vi "Agilent VNA Fetch Data.vi"(4 "Trace":i8=1 min=1 max=99 step=1, 6 "Channel":i8=1 min=1 max=99 step=1, 7 "Agilent VNA":T2, 8 "error in (no error)":errorcluster, 9 "Formatted Data?":bool, 10 "Data to Read (Data)":enum16{"Data", "Memory"}(ring), 11 "VISA Resource Name":refnum<visa-resource-name>) -> (0 "error out":errorcluster, 1 "Display Format":T1, 2 "Data (real+imag)":cdb[](array[numeric]), 3 "dup VISA Resource Name":refnum<visa-resource-name>)   [LabVIEW 2011]
doc: "It is recommended that you hold off triggers before running this VI as the HP8753 tends to \"hang\" if data is read while measurements are being taken.\n\n This VI is used to collect and display data generated by the HP8753 Network Analyzer. The VI can display error-corrected data, error-corrected trace memory, fully formatted data and memory traces. For further information on these types of data see Processsing Chain figure in the HPIB programming note. When the data type is a formatted data, the instruments screen will change to reflect what is being displayed, eg. selecting \"formatted memory\" changes the display to \"MEMORY\".\n\n The data values shown depend upon the data type and the measurement format. If the data type is \"error-corrected data\" or \"error-corrected trace memory\" and/or the measurement format is \"Smith chart\" or \"polar\", the data values are real,imaginary pairs. Otherwise the data values are stimulus,response pairs. These pairs correspond to what is shown in the graphical display.\n\n Data can also be saved to a file with this VI. When saving a file, the stimulus is always shown. The real,imaginary components or the response value are also shown depending upon the data type and the measurement format. \n\n No units are shown on the VI front panel or in the data file. All units are basic units of Hz, dB, seconds, ohms, etc. The \"saved data comments\" control should be used for any special information such as the measurement format, averaging and smoothing information, etc.\n\n Whether or not data is saved and whether the output is in real,imaginary pairs or stimulus,response parirs affects the speed of this VI. When data is saved to a file and/or when data is in stimulus,response pairs, requires the reading of the stimulus values which slows the VI down. The fastest reads are done when the data type is \"error-corrected data\" or \"error-corrected trace memory\" and/or the measurement format is \"Smith chart\" or \"polar\" and data is not being saved to a file.\n\n This VI sets the format, ie. linear or logarithmic, depending upon the sweep type. \n\nFYI - Originally this VI was written without considering the stimulus values. In most case this would be fine for display purposes as the point number could be used for the X value as most sweeps are evenly spaced. This is not the case with frequency list sweeps which can have big gaps in the sweep. For this reason the stimulus value is read (at least in the cases explained above) to make the LabVIEW display match what is display on the instrument's display."
uses:
  TypeDefs/Agilent VNA Instrument Info.ctl
  tests/S Parameter/TypeDefs/SP Measurement Format.ctl
panel:
  out "#data points":i16
  out "bytes to read\n(divide this number\nby 6 bytes per point\nto get # points for\na sanity check)":i16
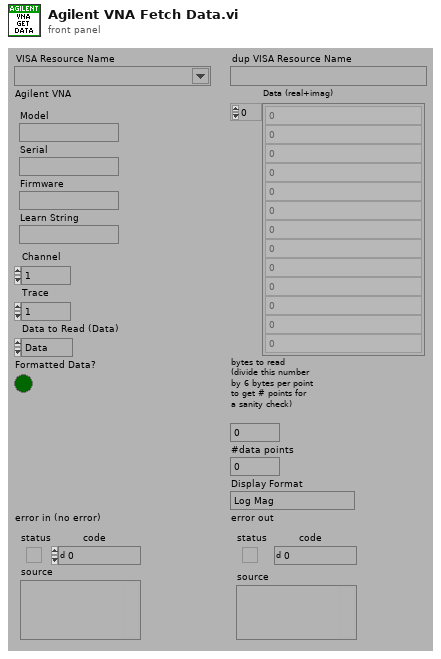
[diagram p1: front panel]
types:
  T1 = typedef "SP Measurement Format.ctl" = enum32{"Log Mag", "Phase", "Delay", "Smith (R+jX)", "Polar (Re/Im)", "Linear Mag", "SWR", "Real", "Imaginary", "Smith (Lin/Phase)", "Smith (Log/Phase)", "Smith (Real/Imag)", "Smith (G+jB)", "Polar (Lin/Phase)", "Polar (Log/Phase)", "Expanded Phase", "Positive Phase", "Inverted Smith", "Unwrapped Phase", "Power Out", "Power In", "Linear Mag/Phase", "Log Mag/Phase", "Real/Imaginary"}
  T2 = typedef "Agilent VNA Instrument Info.ctl" = cluster{"Model":string, "Serial":string, "Firmware":string, "Learn String":string}
  T3 = typedef "Agilent VNA Model.ctl" = enum16{"Not Supported", "8510X", "8719X", "8720X", "8722X", "8753X", "ENA", "PNA", "Field Fox"}
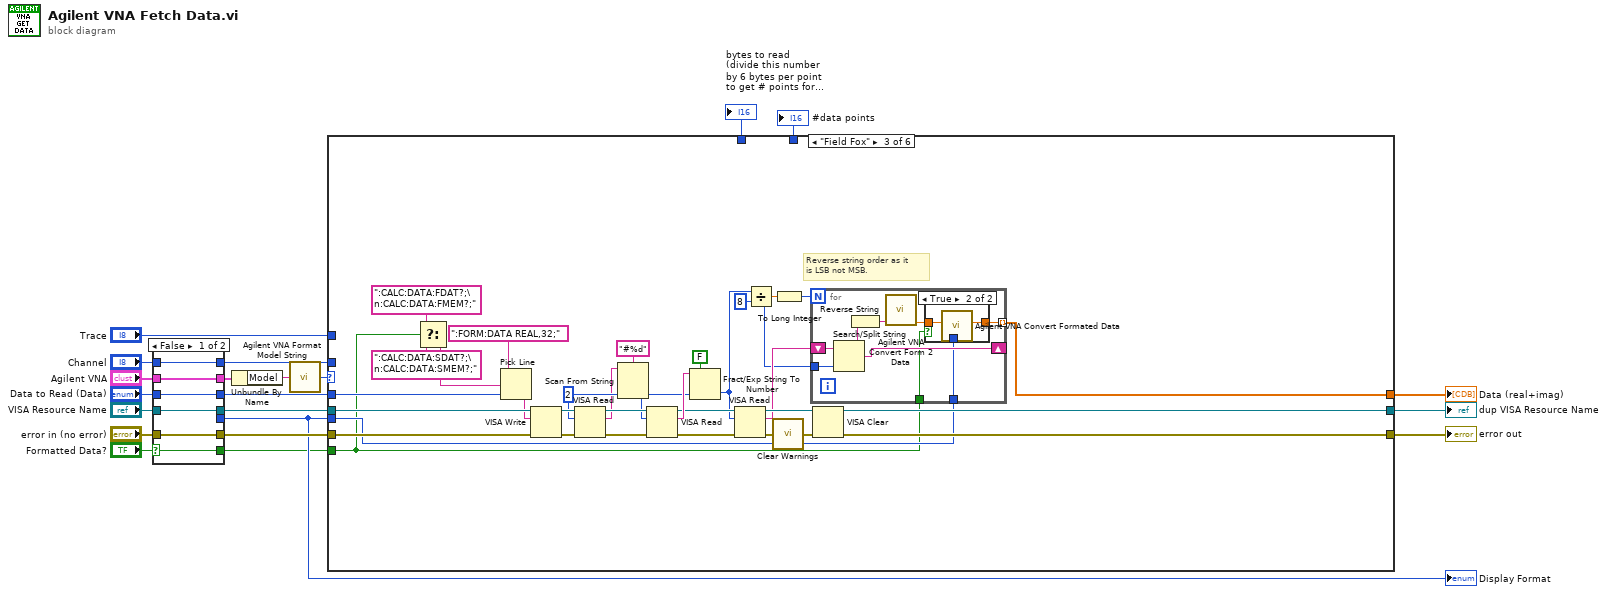
[diagram p0: block diagram]
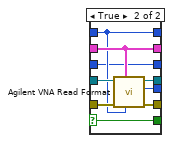
[diagram p2: hidden frame]
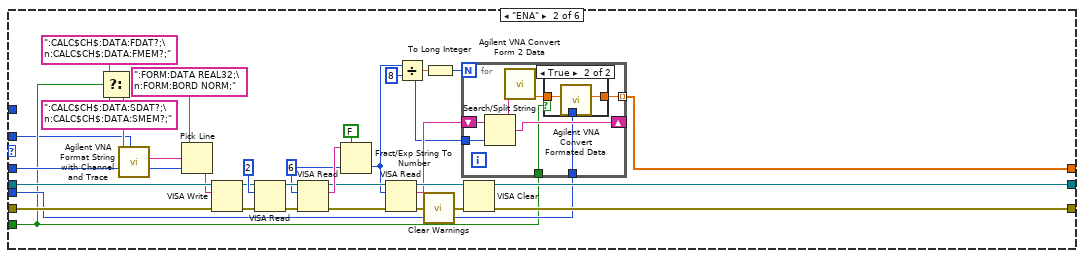
[diagram p4: hidden frame]
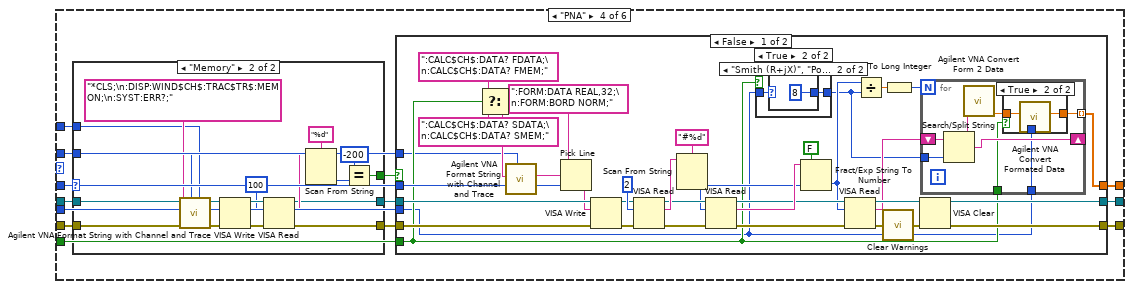
[diagram p7: hidden frame]
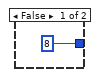
[diagram p9: hidden frame]
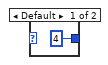
[diagram p10: hidden frame]
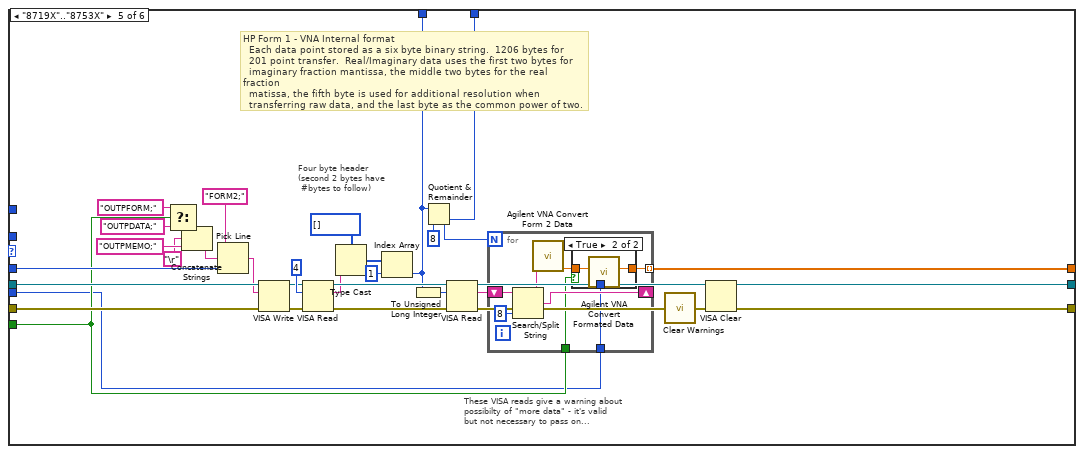
[diagram p13: hidden frame]
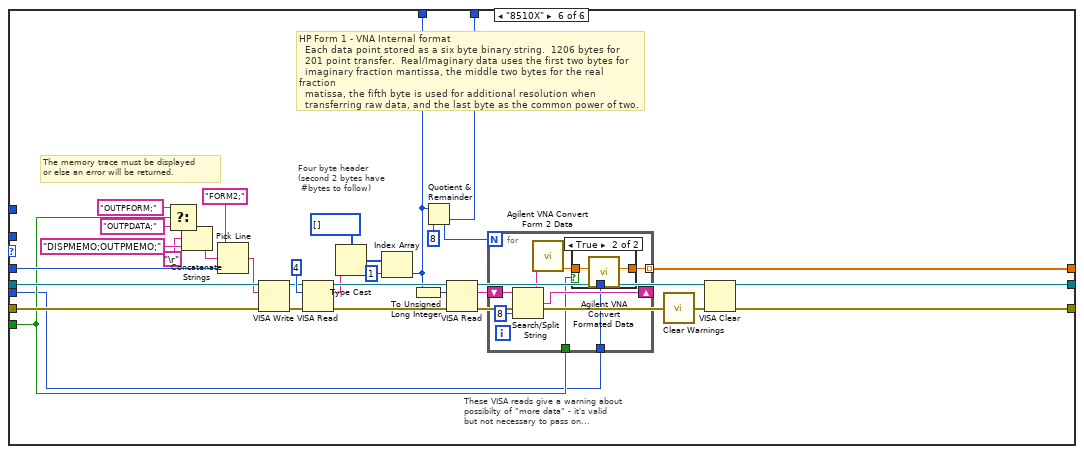
[diagram p15: hidden frame]
diagram:
  n1 = case shown="False" "Formatted Data?" {
    selector: "Formatted Data?" -> [w22 w28]
    tunnel: "error in (no error)" -> [w27 w36]
    tunnel: "VISA Resource Name" -> [w26 w35]
    tunnel: [w26 w34] -> w16
    tunnel: [w27 w33] -> w15
    tunnel: "Agilent VNA" -> [w25 w32]
    tunnel: "Channel" -> [w24 w31]
    tunnel: [w25 w32] -> w2
    tunnel: [w24 w31] -> w12
    tunnel: "Data to Read (Data)" -> [w23 w30]
    tunnel: [w23 w30] -> w10
    tunnel: [_ w29] -> w9
    tunnel: [w22 w28] -> w7
    frame False {
    }
    frame True {
      n2 = call "Agilent VNA Read Format.vi"("Channel"=w31, "Agilent VNA"=w32, "error in (no error)"=w36, "VISA Resource Name"=w35) -> ("error out"=w33:errorcluster, "Display Format"=w29:T1, "dup VISA Resource Name"=w34:refnum<visa-resource-name>)  [unwired: 5 out]
    }
  }
  "Display Format" <- w9
  n3 = Unbundle By Name(w2) -> ("Model"=w1:string)
  n4 = call "Agilent VNA Format Model String.vi"("Model"=w1) -> ("Model"=w19:T3)
  n5 = case shown="\"Field Fox\"" w19 {
    tunnel: w16 -> [w38 w70 w116 w137 w244 w289]
    tunnel: w15 -> [w37 w68 w114 w136 w240 w285]
    tunnel: [w37 w54 w108 w141 w216 w262] -> w3
    tunnel: [_ w48 w107 w140 w224 w269] -> w21
    tunnel: [w38 w55 w109 w142 w217 w261] -> w20
    tunnel: w10 -> [_ w58 w110 w133 w235 w280]
    tunnel: w12 -> [_ w41 _ w132 _ _]
    tunnel: w9 -> [_ w44 w104 w138 w222 w267]
    tunnel: w7 -> [_ w43 w103 w139 w223 w268]
    tunnel: [_ _ _ _ w220 w266] -> w6
    tunnel: [_ _ _ _ w221 w265] -> w5
    tunnel: "Trace" -> [_ _ _ w130 _ _]
    frame "Not Supported" {
    }
    frame "ENA" {
      w42 = 8
      w59 = u32 6
      n6 = Select(t=":CALC$CH$:DATA:FDAT?;\n:CALC$CH$:DATA:FMEM?;" ("String"), s=w43, f=":CALC$CH$:DATA:SDAT?;\n:CALC$CH$:DATA:SMEM?;" ("String")) -> (s? t:f=w45:string)
      n7 = call "Agilent VNA Format String with Channel and Trace.vi"("Channel"=w41, "String"=w45) -> ("String Out"=w66:string)  [unwired: 1 in, 6 out]
      n8 = Pick Line(string ("")=":FORM:DATA REAL32;\n:FORM:BORD NORM;" ("String"), multi-line string=w66, line index=w58) -> (output string=w64:string)
      n9 = VISA Write(VISA resource name=w70, write buffer=w64, error in (no error)=w68) -> (VISA resource name out=w69:refnum<visa-resource-name>, error out=w67:errorcluster)  [unwired: 1 out]
      n10 = VISA Read(VISA resource name=w69, byte count=u32 2, error in (no error)=w67) -> (VISA resource name out=w63:refnum<visa-resource-name>, error out=w62:errorcluster)  [unwired: 2 out]
      n11 = VISA Read(VISA resource name=w63, byte count=w59, error in (no error)=w62) -> (VISA resource name out=w53:refnum<visa-resource-name>, read buffer=w60:string, error out=w52:errorcluster)  [unwired: 1 out]
      n12 = Fract/Exp String To Number(use system decimal point (T)=FALSE, string=w60, default (0 dbl)=w59) -> (number=w51:u32)  [unwired: 2 out]
      n13 = VISA Read(VISA resource name=w53, byte count=w51, error in (no error)=w52) -> (VISA resource name out=w50:refnum<visa-resource-name>, read buffer=w49:string, error out=w40:errorcluster)  [unwired: 1 out]
      n14 = Divide(x=w51, y=w42) -> (x/y=w57:dbl)
      n15 = call "Clear Warnings.vi"("error in (no error)"=w40) -> ("error out"=w39:errorcluster)
      n16 = To Long Integer(number=w57) -> (32bit integer=w56:i32)
      n17 = for {
        N: w56 -> [_]
        shift-right: [w77] -> _
        shift-left: w49 -> [w78]
        tunnel: [w75] -> w48 mode=indexing
        tunnel: w44 -> [w74]
        tunnel: w43 -> [w73]
        tunnel: w42 -> [w72]
        n18 = Search/Split String(string=w78, offset (0)=w72) -> (substring before match=w76:string, match + rest of string=w77:string)  [unwired: 2 out]
        n19 = call "Agilent VNA Convert Form 2 Data.vi"("Raw Data Point"=w76) -> ("Number"=w79:cdb)  [unwired: 10 out]
        n20 = case shown="True" w73 {
          tunnel: w79 -> [w80 w82]
          tunnel: [w80 w81] -> w75
          tunnel: w74 -> [_ w83]
          frame False {
          }
          frame True {
            n21 = call "Agilent VNA Convert Formated Data.vi"("Display Format"=w83, "Number"=w82) -> ("Number"=w81:cdb)  [unwired: 9 out]
          }
        }
      }
      n22 = VISA Clear(VISA resource name=w50, error in (no error)=w39) -> (VISA resource name out=w55:refnum<visa-resource-name>, error out=w54:errorcluster)
    }
    frame "Field Fox" {
      w91 = 8
      w86 = u32 2
      # "Reverse string order as it\nis LSB not MSB."
      n23 = Select(t=":CALC:DATA:FDAT?;\n:CALC:DATA:FMEM?;" ("String"), s=w103, f=":CALC:DATA:SDAT?;\n:CALC:DATA:SMEM?;" ("String")) -> (s? t:f=w102:string)
      n24 = Pick Line(string ("")=":FORM:DATA REAL,32;" ("String"), multi-line string=w102, line index=w110) -> (output string=w111:string)
      n25 = VISA Write(VISA resource name=w116, write buffer=w111, error in (no error)=w114) -> (VISA resource name out=w115:refnum<visa-resource-name>, error out=w113:errorcluster)  [unwired: 1 out]
      n26 = VISA Read(VISA resource name=w115, byte count=w86, error in (no error)=w113) -> (VISA resource name out=w101:refnum<visa-resource-name>, read buffer=w84:string, error out=w100:errorcluster)  [unwired: 1 out]
      n27 = Scan From String(format string="#%d", input string=w84, default 1=w86) -> (output 1=w85:u32)  [unwired: 2 in, 3 out]
      n28 = VISA Read(VISA resource name=w101, byte count=w85, error in (no error)=w100) -> (VISA resource name out=w96:refnum<visa-resource-name>, read buffer=w99:string, error out=w95:errorcluster)  [unwired: 1 out]
      n29 = Fract/Exp String To Number(use system decimal point (T)=FALSE, string=w99, default (0 dbl)=w85) -> (number=w94:u32)  [unwired: 2 out]
      n30 = VISA Read(VISA resource name=w96, byte count=w94, error in (no error)=w95) -> (VISA resource name out=w93:refnum<visa-resource-name>, read buffer=w92:string, error out=w90:errorcluster)  [unwired: 1 out]
      n31 = Divide(x=w94, y=w91) -> (x/y=w98:dbl)
      n32 = call "Clear Warnings.vi"("error in (no error)"=w90) -> ("error out"=w89:errorcluster)
      n33 = To Long Integer(number=w98) -> (32bit integer=w97:i32)
      n34 = for {
        N: w97 -> [_]
        shift-right: [w123] -> _
        shift-left: w92 -> [w124]
        tunnel: [w122] -> w107 mode=indexing
        tunnel: w104 -> [w121]
        tunnel: w103 -> [w120]
        tunnel: w91 -> [w119]
        n35 = Search/Split String(string=w124, offset (0)=w119) -> (substring before match=w118:string, match + rest of string=w123:string)  [unwired: 2 out]
        n36 = Reverse String(1:w118) -> (0:w117:string)
        n37 = call "Agilent VNA Convert Form 2 Data.vi"("Raw Data Point"=w117) -> ("Number"=w125:cdb)  [unwired: 10 out]
        n38 = case shown="True" w120 {
          tunnel: w125 -> [w126 w128]
          tunnel: [w126 w127] -> w122
          tunnel: w121 -> [_ w129]
          frame False {
          }
          frame True {
            n39 = call "Agilent VNA Convert Formated Data.vi"("Display Format"=w129, "Number"=w128) -> ("Number"=w127:cdb)  [unwired: 9 out]
          }
        }
      }
      n40 = VISA Clear(VISA resource name=w93, error in (no error)=w89) -> (VISA resource name out=w109:refnum<visa-resource-name>, error out=w108:errorcluster)
    }
    frame "PNA" {
      n41 = case shown="\"Memory\"" w133 {
        tunnel: w137 -> [w144 w160]
        tunnel: w136 -> [w143 w159]
        tunnel: [w144 w151] -> w135
        tunnel: [w143 w150] -> w134
        tunnel: w132 -> [_ w146]
        tunnel: [_ w147] -> w131
        tunnel: w130 -> [_ w145]
        frame "Data", Default {
        }
        frame "Memory" {
          n42 = call "Agilent VNA Format String with Channel and Trace.vi"("Trace"=w145, "Channel"=w146, "String"="*CLS;\n:DISP:WIND$CH$:TRAC$TR$:MEM ON;\n:SYST:ERR?;") -> ("String Out"=w157:string)  [unwired: 6 out]
          n43 = VISA Write(VISA resource name=w160, write buffer=w157, error in (no error)=w159) -> (VISA resource name out=w156:refnum<visa-resource-name>, error out=w155:errorcluster)  [unwired: 1 out]
          n44 = VISA Read(VISA resource name=w156, byte count=u32 100, error in (no error)=w155) -> (VISA resource name out=w151:refnum<visa-resource-name>, read buffer=w153:string, error out=w150:errorcluster)  [unwired: 1 out]
          n45 = Scan From String(format string="%d", input string=w153) -> (output 1=w149:i32)  [unwired: 2 in, 4 out]
          n46 = Equal?(x=-200, y=w149) -> (x = y?=w147:bool)
        }
      }
      n47 = case shown="False" w131 {
        tunnel: w135 -> [w194 w213]
        tunnel: w134 -> [w192 w214]
        tunnel: w133 -> [w185 _]
        tunnel: [w182 w213] -> w142
        tunnel: [w181 w214] -> w141
        tunnel: w132 -> [w163 _]
        tunnel: [w175 _] -> w140
        tunnel: w139 -> [w166 _]
        tunnel: w138 -> [w165 _]
        frame False {
          n48 = Select(t=":CALC$CH$:DATA? FDATA;\n:CALC$CH$:DATA? FMEM;" ("String"), s=w166, f=":CALC$CH$:DATA? SDATA;\n:CALC$CH$:DATA? SMEM;" ("String")) -> (s? t:f=w172:string)
          n49 = call "Agilent VNA Format String with Channel and Trace.vi"("Channel"=w163, "String"=w172) -> ("String Out"=w190:string)  [unwired: 1 in, 6 out]
          n50 = Pick Line(string ("")=":FORM:DATA REAL,32;\n:FORM:BORD NORM;" ("String"), multi-line string=w190, line index=w185) -> (output string=w188:string)
          n51 = VISA Write(VISA resource name=w194, write buffer=w188, error in (no error)=w192) -> (VISA resource name out=w193:refnum<visa-resource-name>, error out=w191:errorcluster)  [unwired: 1 out]
          n52 = VISA Read(VISA resource name=w193, byte count=u32 2, error in (no error)=w191) -> (VISA resource name out=w168:refnum<visa-resource-name>, read buffer=w171:string, error out=w169:errorcluster)  [unwired: 1 out]
          n53 = Scan From String(format string="#%d", input string=w171) -> (output 1=w167:i32)  [unwired: 2 in, 4 out]
          n54 = VISA Read(VISA resource name=w168, byte count=w167, error in (no error)=w169) -> (VISA resource name out=w180:refnum<visa-resource-name>, read buffer=w186:string, error out=w179:errorcluster)  [unwired: 1 out]
          n55 = case shown="True" w166 {
            tunnel: w165 -> [_ w198]
            tunnel: [8 w197] -> w164
            frame False {
            }
            frame True {
              n56 = case shown="\"Smith (R+jX)\", \"Polar (Re/Im)\", \"Smith (Lin/Phase)\"..\"Polar (Log/Phase)\", \"Inverted Smith\"" w198 {
                tunnel: [4 8] -> w197
                frame Default {
                }
                frame "Smith (R+jX)", "Polar (Re/Im)", "Smith (Lin/Phase)".."Polar (Log/Phase)", "Inverted Smith" {
                }
              }
            }
          }
          n57 = Fract/Exp String To Number(use system decimal point (T)=FALSE, string=w186, default (0 dbl)=w167) -> (number=w178:i32)  [unwired: 2 out]
          n58 = VISA Read(VISA resource name=w180, byte count=w178, error in (no error)=w179) -> (VISA resource name out=w177:refnum<visa-resource-name>, read buffer=w176:string, error out=w162:errorcluster)  [unwired: 1 out]
          n59 = Divide(x=w178, y=w164) -> (x/y=w184:dbl)
          n60 = call "Clear Warnings.vi"("error in (no error)"=w162) -> ("error out"=w161:errorcluster)
          n61 = To Long Integer(number=w184) -> (32bit integer=w183:i32)
          n62 = VISA Clear(VISA resource name=w177, error in (no error)=w161) -> (VISA resource name out=w182:refnum<visa-resource-name>, error out=w181:errorcluster)
          n63 = for {
            N: w183 -> [_]
            shift-right: [w206] -> _
            shift-left: w176 -> [w207]
            tunnel: [w204] -> w175 mode=indexing
            tunnel: w165 -> [w203]
            tunnel: w166 -> [w202]
            tunnel: w164 -> [w201]
            n64 = Search/Split String(string=w207, offset (0)=w201) -> (substring before match=w205:string, match + rest of string=w206:string)  [unwired: 2 out]
            n65 = call "Agilent VNA Convert Form 2 Data.vi"("Raw Data Point"=w205) -> ("Number"=w208:cdb)  [unwired: 10 out]
            n66 = case shown="True" w202 {
              tunnel: w208 -> [w209 w211]
              tunnel: [w209 w210] -> w204
              tunnel: w203 -> [_ w212]
              frame False {
              }
              frame True {
                n67 = call "Agilent VNA Convert Formated Data.vi"("Display Format"=w212, "Number"=w211) -> ("Number"=w210:cdb)  [unwired: 9 out]
              }
            }
          }
        }
        frame True {
        }
      }
    }
    frame "8719X".."8753X" {
      # "These VISA reads give a warning about\npossibilty of \"more data\" - it's valid\nbut not necessary to pass on..."
      # "Four byte header\n(second 2 bytes have\n #bytes to follow)"
      # "HP Form 1 - VNA Internal format\n  Each data point stored as a six byte binary string.  1206 bytes for\n  201 point transfer.  Real/Imaginary data uses the first two bytes for\n  imaginary fraction mantissa, the middle two bytes for the real fraction\n  matissa, the fifth byte is used for additional resolution when\n  transferring raw data, and the last byte as the common power of two."
      n68 = Select(t="OUTPFORM;", s=w223, f="OUTPDATA;") -> (s? t:f=w226:string)
      n69 = Concatenate Strings(w226, "\r", "OUTPMEMO;") -> (w230:string)
      n70 = Pick Line(string ("")="FORM2;", multi-line string=w230, line index=w235) -> (output string=w234:string)
      n71 = VISA Write(VISA resource name=w244, write buffer=w234, error in (no error)=w240) -> (VISA resource name out=w233:refnum<visa-resource-name>, error out=w232:errorcluster)  [unwired: 1 out]
      n72 = VISA Read(VISA resource name=w233, byte count=u32 4, error in (no error)=w232) -> (VISA resource name out=w246:refnum<visa-resource-name>, read buffer=w238:string, error out=w245:errorcluster)  [unwired: 1 out]
      n73 = Type Cast(type=i16[] [], x=w238) -> (*(type *) &x=w237:i16[])
      n74 = Index Array(array=w237, index=1) -> (element=w221:i16)
      n75 = To Unsigned Long Integer(number=w221) -> (unsigned 32bit integer=w242:u32)
      n76 = Quotient & Remainder(x=w221, y=i16 8) -> (floor(x/y)=w220:i16)  [unwired: 1 out]
      n77 = VISA Read(VISA resource name=w246, byte count=w242, error in (no error)=w245) -> (VISA resource name out=w219:refnum<visa-resource-name>, read buffer=w239:string, error out=w215:errorcluster)  [unwired: 1 out]
      n78 = for {
        N: w220 -> [_]
        shift-right: [w254] -> _
        shift-left: w239 -> [w255]
        tunnel: [w250] -> w224 mode=indexing
        tunnel: w223 -> [w249]
        tunnel: w222 -> [w248]
        n79 = Search/Split String(string=w255, offset (0)=8) -> (substring before match=w252:string, match + rest of string=w254:string)  [unwired: 2 out]
        n80 = call "Agilent VNA Convert Form 2 Data.vi"("Raw Data Point"=w252) -> ("Number"=w251:cdb)  [unwired: 10 out]
        n81 = case shown="True" w249 {
          tunnel: w251 -> [w256 w258]
          tunnel: [w256 w257] -> w250
          tunnel: w248 -> [_ w259]
          frame False {
          }
          frame True {
            n82 = call "Agilent VNA Convert Formated Data.vi"("Display Format"=w259, "Number"=w258) -> ("Number"=w257:cdb)  [unwired: 9 out]
          }
        }
      }
      n83 = call "Clear Warnings.vi"("error in (no error)"=w215) -> ("error out"=w218:errorcluster)
      n84 = VISA Clear(VISA resource name=w219, error in (no error)=w218) -> (VISA resource name out=w217:refnum<visa-resource-name>, error out=w216:errorcluster)
    }
    frame "8510X" {
      # "The memory trace must be displayed\nor else an error will be returned."
      # "These VISA reads give a warning about\npossibilty of \"more data\" - it's valid\nbut not necessary to pass on..."
      # "Four byte header\n(second 2 bytes have\n #bytes to follow)"
      # "HP Form 1 - VNA Internal format\n  Each data point stored as a six byte binary string.  1206 bytes for\n  201 point transfer.  Real/Imaginary data uses the first two bytes for\n  imaginary fraction mantissa, the middle two bytes for the real fraction\n  matissa, the fifth byte is used for additional resolution when\n  transferring raw data, and the last byte as the common power of two."
      n85 = Select(t="OUTPFORM;", s=w268, f="OUTPDATA;") -> (s? t:f=w271:string)
      n86 = Concatenate Strings(w271, "\r", "DISPMEMO;OUTPMEMO;") -> (w275:string)
      n87 = Pick Line(string ("")="FORM2;", multi-line string=w275, line index=w280) -> (output string=w279:string)
      n88 = VISA Write(VISA resource name=w289, write buffer=w279, error in (no error)=w285) -> (VISA resource name out=w278:refnum<visa-resource-name>, error out=w277:errorcluster)  [unwired: 1 out]
      n89 = VISA Read(VISA resource name=w278, byte count=u32 4, error in (no error)=w277) -> (VISA resource name out=w291:refnum<visa-resource-name>, read buffer=w283:string, error out=w290:errorcluster)  [unwired: 1 out]
      n90 = Type Cast(type=i16[] [], x=w283) -> (*(type *) &x=w282:i16[])
      n91 = Index Array(array=w282, index=1) -> (element=w265:i16)
      n92 = To Unsigned Long Integer(number=w265) -> (unsigned 32bit integer=w287:u32)
      n93 = Quotient & Remainder(x=w265, y=i16 8) -> (floor(x/y)=w266:i16)  [unwired: 1 out]
      n94 = VISA Read(VISA resource name=w291, byte count=w287, error in (no error)=w290) -> (VISA resource name out=w263:refnum<visa-resource-name>, read buffer=w284:string, error out=w260:errorcluster)  [unwired: 1 out]
      n95 = for {
        N: w266 -> [_]
        shift-right: [w299] -> _
        shift-left: w284 -> [w300]
        tunnel: [w295] -> w269 mode=indexing
        tunnel: w268 -> [w294]
        tunnel: w267 -> [w293]
        n96 = Search/Split String(string=w300, offset (0)=8) -> (substring before match=w297:string, match + rest of string=w299:string)  [unwired: 2 out]
        n97 = call "Agilent VNA Convert Form 2 Data.vi"("Raw Data Point"=w297) -> ("Number"=w296:cdb)  [unwired: 10 out]
        n98 = case shown="True" w294 {
          tunnel: w296 -> [w301 w303]
          tunnel: [w301 w302] -> w295
          tunnel: w293 -> [_ w304]
          frame False {
          }
          frame True {
            n99 = call "Agilent VNA Convert Formated Data.vi"("Display Format"=w304, "Number"=w303) -> ("Number"=w302:cdb)  [unwired: 9 out]
          }
        }
      }
      n100 = call "Clear Warnings.vi"("error in (no error)"=w260) -> ("error out"=w264:errorcluster)
      n101 = VISA Clear(VISA resource name=w263, error in (no error)=w264) -> (VISA resource name out=w261:refnum<visa-resource-name>, error out=w262:errorcluster)
    }
  }
  "dup VISA Resource Name" <- w20
  "error out" <- w3
  "Data (real+imag)" <- w21
  "bytes to read\n(divide this number\nby 6 bytes per point\nto get # points for\na sanity check)" <- w5
  "#data points" <- w6
